vi "New Current Value Table.vi"(8 "error in (no error)":errorcluster) -> (0 "error out":errorcluster, 3 "Current Value Table":T1)   [LabVIEW 2015, in "CurrentValueTable.lvlib" / "CurrentValueTable.lvclass"]
uses:
  CurrentValueTable.lvclass
  CurrentValueTable Reference.ctl
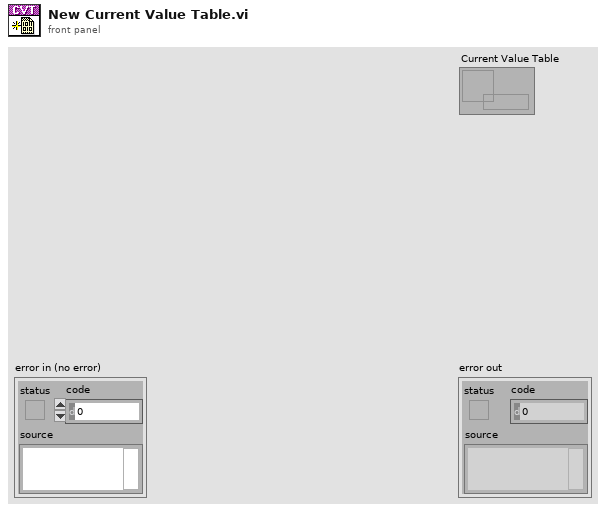
[diagram p1: front panel]
types:
  T1 = typedef "CurrentValueTable.lvlib/CurrentValueTable.lvclass/CurrentValueTable Reference.ctl" = refnum<data-value>
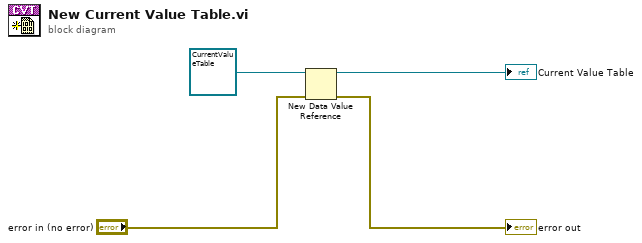
[diagram p0: block diagram]
diagram:
  n1 = New Data Value Reference(data value=refnum<class "CurrentValueTable.lvclass"> refnum ("CurrentValueTable in"), error in="error in (no error)") -> (data value reference=→"Current Value Table":refnum<data-value>, error out=→"error out":errorcluster)
